vi "Untitled 1.vi"() -> ()   [LabVIEW 2010]
panel:
  out "length 2":i32
  out "length":i32
  out "x/y":dbl=4.0
  in  "String":string="<?xml version=\"1.0\" encoding=\"UTF-8\"?>\n<methodCall>\n\t<methodName>jil.syncvi</methodName>\n<params>\n  <param>\n    <value>\n    <array>\n\n      <value>\n      <struct>\n        <member>\n          <name>name</name>\n          <value><string>intin</string></value>\n        </member>\n        <member>\n          <name>action</name>\n          <value><string>set</string></value>\n        </member>\n        <member>\n          <name>value</name>\n          <value><int>0</int></value>\n        </member>\n      </struct>\n      </value>\n\n\n      <value>\n      <struct>\n        <member>\n          <name>name</name>\n          <value><string>doublein</string></value>\n        </member>\n        <member>\n          <name>action</name>\n          <value><string>set</string></value>\n        </member>\n        <member>\n          <name>value</name>\n          <value><double>0,000000</double></value>\n        </member>\n      </struct>\n      </value>\n\n      <value>\n      <struct>\n        <member>\n          <name>name</name>\n          <value><string>booleanin</string></value>\n        </member>\n        <member>\n          <name>action</name>\n          <value><string>set</string></value>\n        </member>\n        <member>\n          <name>value</name>\n          <value><boolean>1</boolean></value>\n        </member>\n      </struct>\n      </value>\n\n      <value>\n      <struct>\n        <member>\n          <name>name</name>\n          <value><string>stringin</string></value>\n        </member>\n        <member>\n          <name>action</name>\n          <value><string>set</string></value>\n        </member>\n        <member>\n          <name>value</name>\n          <value><string></string></value>\n        </member>\n      </struct>\n      </value>\n\n\n      <value>\n      <struct>\n        <member>\n          <name>name</name>\n          <value><string>intout</string></value>\n        </member>\n        <member>\n          <name>action</name>\n          <value><string>get</string></value>\n        </member>\n        <member>\n          <name>value</name>\n          <value><int>0</int></value>\n        </member>\n      </struct>\n      </value>\n\n\n      <value>\n      <struct>\n        <member>\n          <name>name</name>\n          <value><string>doubleout</string></value>\n        </member>\n        <member>\n          <name>action</name>\n          <value><string>get</string></value>\n        </member>\n        <member>\n          <name>value</name>\n          <value><double>0</double></value>\n        </member>\n      </struct>\n      </value>\n\n      <value>\n      <struct>\n        <member>\n          <name>name</name>\n          <value><string>booleanout</string></value>\n        </member>\n        <member>\n          <name>action</name>\n          <value><string>get</string></value>\n        </member>\n        <member>\n          <name>value</name>\n          <value><boolean>0</boolean></value>\n        </member>\n      </struct>\n      </value>\n\n      <value>\n      <struct>\n        <member>\n          <name>name</name>\n          <value><string>stringout</string></value>\n        </member>\n        <member>\n          <name>action</name>\n          <value><string>get</string></value>\n        </member>\n        <member>\n          <name>value</name>\n          <value><string>a</string></value>\n        </member>\n      </struct>\n      </value>\n\n\n    </array>\n    </value>\n  </param>\n</params>\n</methodCall>"
  out "error out":errorcluster
  out "Uncompressed String":string="hola esto es una pruena a ver que tal"
  out "GZIP compressed string":string
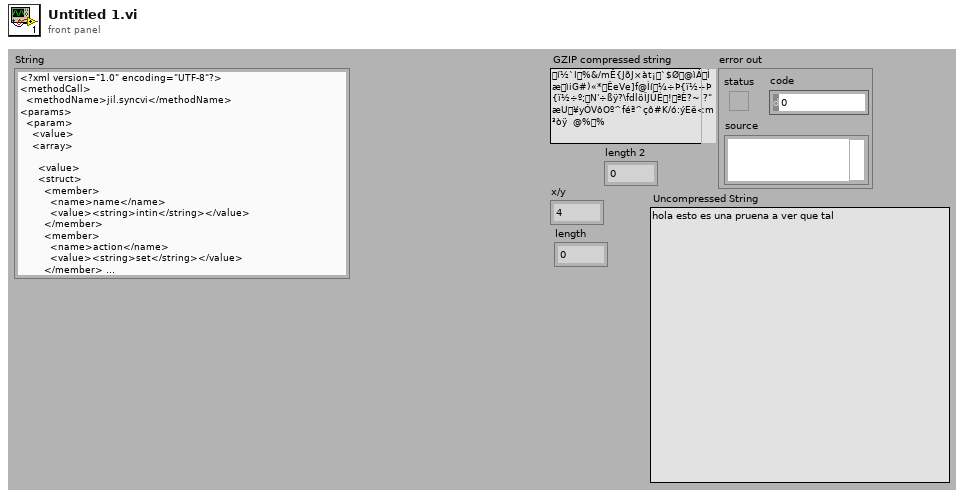
[diagram p1: front panel]
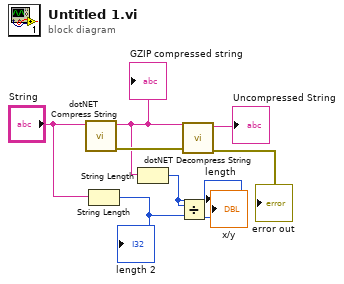
[diagram p0: block diagram]
diagram:
  n1 = call "dotNET Compress String.vi"("String"="String") -> ("error out"=w7:errorcluster, "GZIP compressed string"=w4:string)  [unwired: 8 in, 1 out]
  "GZIP compressed string" <- w4
  n2 = String Length(string="String") -> (length=w1:i32)
  "length 2" <- w1
  n3 = String Length(string=w4) -> (length=w2:i32)
  "length" <- w2
  n4 = Divide(x=w2, y=w1) -> (x/y=→"x/y":dbl)
  n5 = call "dotNET Decompress String.vi"("error in (no error)"=w7, "GZIP Compressed String"=w4) -> ("error out"=→"error out":errorcluster, "Uncompressed String"=→"Uncompressed String":string)  [unwired: 8 in]
